vi "Init Task.vi"(4 "counter":tag, 6 "line grouping":i32(ring) items=["one channel for each line", "one channel for all lines"], 7 "physical channels":tag, 8 "error in (no error)":errorcluster, 9 "name":string, 10 "DAQmxTaksContainer_General IN":refnum<class "DAQmxTaksContainer_General.lvclass">, 11 "DAQmxTaskAITension in":refnum<class "DAQmxTaskAIVoltage.lvclass">) -> (0 "error out":errorcluster, 3 "DAQmxTaskAITension out":refnum<class "DAQmxTaskAIVoltage.lvclass">)   [LabVIEW 2018, in "DAQmxTaskAIVoltage.lvclass"]
uses:
  DAQmxTaskAIVoltage.lvclass
  C:/Users/Sergey Denisov/Documents/REPS/TRANCON/Classes/DAQmxTasks/DAQmxTask.lvclass
  DAQmxTaskContainer_General/DAQmxTaksContainer_General.lvclass
  DAQmxTaskContainer_General/DAQmxTaksContainer_General.lvclass/DAQmxTaksContainer_General.ctl
  DAQmxTask.lvclass/DAQmxTask.ctl
  <vilib>/DAQmx/create/channels.llb/DAQmx Create Channel (AI-Voltage-Basic).vi
  DAQmxTask.lvclass
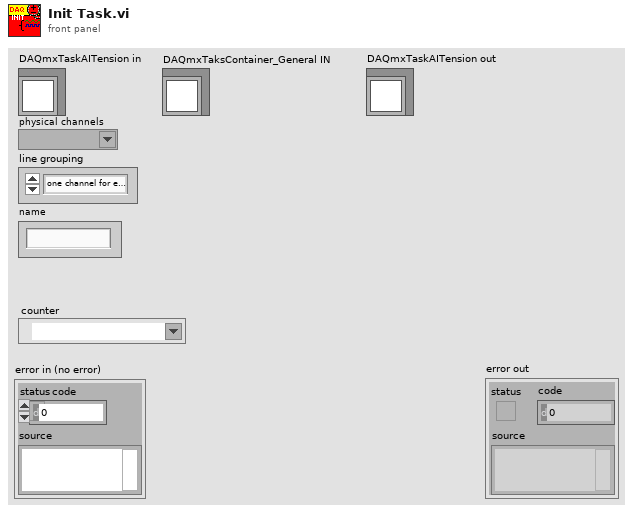
[diagram p1: front panel]
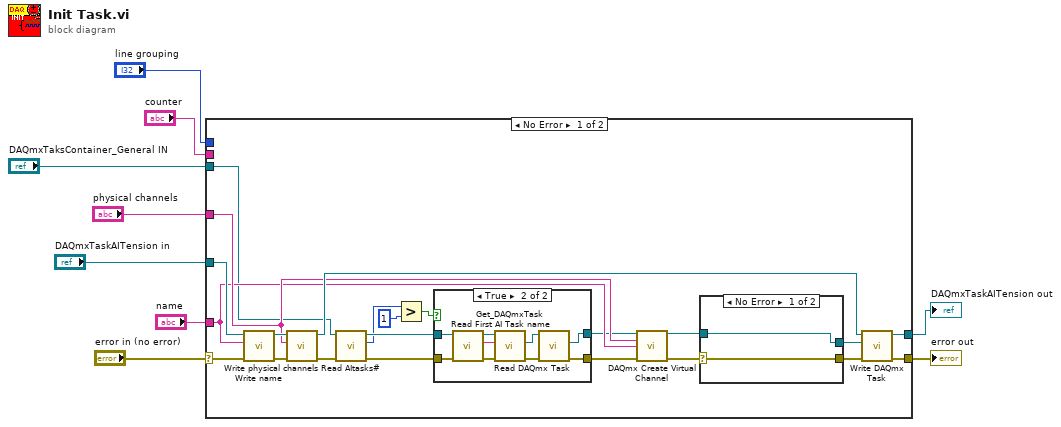
[diagram p0: block diagram]
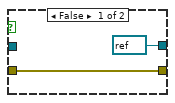
[diagram p2: hidden frame]
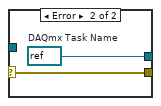
[diagram p3: hidden frame]
diagram:
  n1 = case shown="No Error" "error in (no error)" {
    selector: "error in (no error)" -> [w31 w48]
    tunnel: [w18 w48] -> w6
    tunnel: "name" -> [w21 _]
    tunnel: "physical channels" -> [w27 _]
    tunnel: "DAQmxTaskAITension in" -> [w26 w47]
    tunnel: "counter" -> [_ _]
    tunnel: "line grouping" -> [_ _]
    tunnel: "DAQmxTaksContainer_General IN" -> [w17 _]
    tunnel: [w13 w47] -> w1
    frame No Error {
      n2 = call "Write name.vi"("error in (no error)"=w31, "name"=w21, "DAQmxTask in"=w26) -> ("error out"=w29:errorcluster, "DAQmxTask out"=w30:refnum<class "DAQmxTaskAIVoltage.lvclass">)  [unwired: 7 in]
      n3 = call "Write physical channels.vi"("error in (no error)"=w29, "physical channels"=w27, "DAQmxTask in"=w30) -> ("error out"=w16:errorcluster, "DAQmxTask out"=w28:refnum<class "DAQmxTaskAIVoltage.lvclass">)  [unwired: 7 in]
      n4 = call "Read AItasks#.vi"("error in (no error)"=w16, "DAQmxTaksContainer_General in"=w17) -> ("error out"=w19:errorcluster, "AItasks#"=w12:i32, "DAQmxTaksContainer_General out"=w20:refnum<class "DAQmxTaksContainer_General.lvclass">)  [unwired: 7 in]
      n5 = Greater?(x=w12, y=1) -> (0:w10:bool)
      n6 = case shown="True" w10 {
        tunnel: w20 -> [_ w37]
        tunnel: w19 -> [w33 w38]
        tunnel: [w33 w41] -> w15
        tunnel: [refnum<k21> refnum ("DAQmx Task Name") w34] -> w14
        frame False {
        }
        frame True {
          n7 = call "Read First AI Task name.vi"("error in (no error)"=w38, "DAQmxTaksContainer_General in"=w37) -> ("error out"=w39:errorcluster, "First AI Task name"=w35:string, "DAQmxTaksContainer_General out"=w36:refnum<class "DAQmxTaksContainer_General.lvclass">)  [unwired: 7 in]
          n8 = call "Get_DAQmxTask.vi"("error in (no error)"=w39, "Task name"=w35, "DAQmxTaksContainer_General in"=w36) -> ("error out"=w42:errorcluster, "DAQmx Task"=w40:refnum<class "DAQmxTask.lvclass">)  [unwired: 6 in, 1 out]
          n9 = call "Read DAQmx Task.vi"("error in (no error)"=w42, "DAQmxTask in"=w40) -> ("error out"=w41:errorcluster, "DAQmx Task Name"=w34:refnum<k21>)  [unwired: 7 in, 1 out]
        }
      }
      n10 = call-poly <vilib>:"DAQmx Create Virtual Channel.vi"("task in"=w14, "physical channels"=w27, "name to assign"=w21, "error in"=w15) -> ("task out"=w25:refnum<k21>, "error out"=w24:errorcluster)  [unwired: 10 in]
      n11 = case shown="No Error" w24 {
        selector: w24 -> [w43 w45]
        tunnel: [w44 w46] -> w23
        tunnel: w25 -> [w44 _]
        tunnel: [w43 w45] -> w22
        frame No Error {
        }
        frame Error {
          w46 = refnum<k21> refnum  # DAQmx Task Name
        }
      }
      n12 = call "Write DAQmx Task.vi"("error in (no error)"=w22, "DAQmx Task Name"=w23, "DAQmxTask in"=w28) -> ("error out"=w18:errorcluster, "DAQmxTask out"=w13:refnum<class "DAQmxTaskAIVoltage.lvclass">)  [unwired: 7 in]
    }
    frame Error {
    }
  }
  "error out" <- w6
  "DAQmxTaskAITension out" <- w1
